vi "Name to Path.vi"(10 "Employee Sheets Path":path=path "C:/Users/Voicelab/Desktop/CheckIn/Employee Sheets", 11 "Employee Name":string) -> (3 "Sheet Path":path)   [LabVIEW 2015]
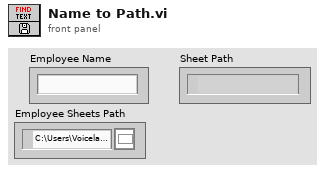
[diagram p1: front panel]
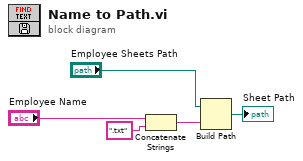
[diagram p0: block diagram]
diagram:
  n1 = Concatenate Strings("Employee Name", ".txt" ("string")) -> (w2:string)
  n2 = Build Path(base path="Employee Sheets Path", name or relative path=w2) -> (appended path=→"Sheet Path":path)
